vi "Create Command String.vi"(8 "error in (no error)":errorcluster, 11 "Channel Params":T1={"channel"=enum."2", "gain"=enum."10x", "input"=enum."DIFF", "shunt"=enum."Open", "couple"=enum."DC", "filter"=enum."ON"}) -> (0 "error out":errorcluster, 3 "Command string":string)   [LabVIEW 2019, in "KH7008.lvlib"]
uses:
  KH7008.lvlib
  typedefs/channelProperties--Cluster.ctl
  typedefs/channel--enum.ctl
  typedefs/gain--enum.ctl
  typedefs/input--enum.ctl
  typedefs/shunt--enum.ctl
  typedefs/couple--enum.ctl
  typedefs/filter--enum.ctl
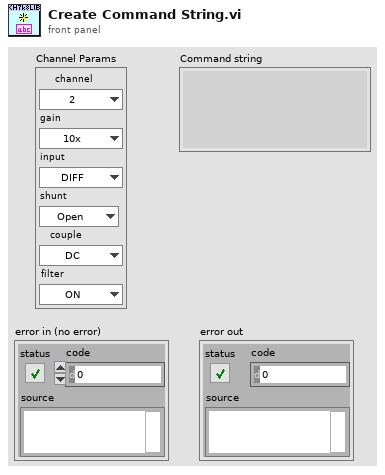
[diagram p1: front panel]
types:
  T1 = typedef "KH7008.lvlib/channelProperties--Cluster.ctl" = cluster{"channel":T2, "gain":T3, "input":T4, "shunt":T5, "couple":T6, "filter":T7}
  T2 = typedef "KH7008.lvlib/channel--enum.ctl" = enum16{"1", "2", "3", "4", "5", "6", "7", "8"}
  T3 = typedef "KH7008.lvlib/gain--enum.ctl" = enum16{"1x", "10x", "100x", "1000x"}
  T4 = typedef "KH7008.lvlib/input--enum.ctl" = enum16{"OFF", "SE+", "SE-", "DIFF"}
  T5 = typedef "KH7008.lvlib/shunt--enum.ctl" = enum16{"Open", "50", "500", "5k", "50k", "10M"}
  T6 = typedef "KH7008.lvlib/couple--enum.ctl" = enum16{"AC", "DC"}
  T7 = typedef "KH7008.lvlib/filter--enum.ctl" = enum16{"OFF", "ON"}
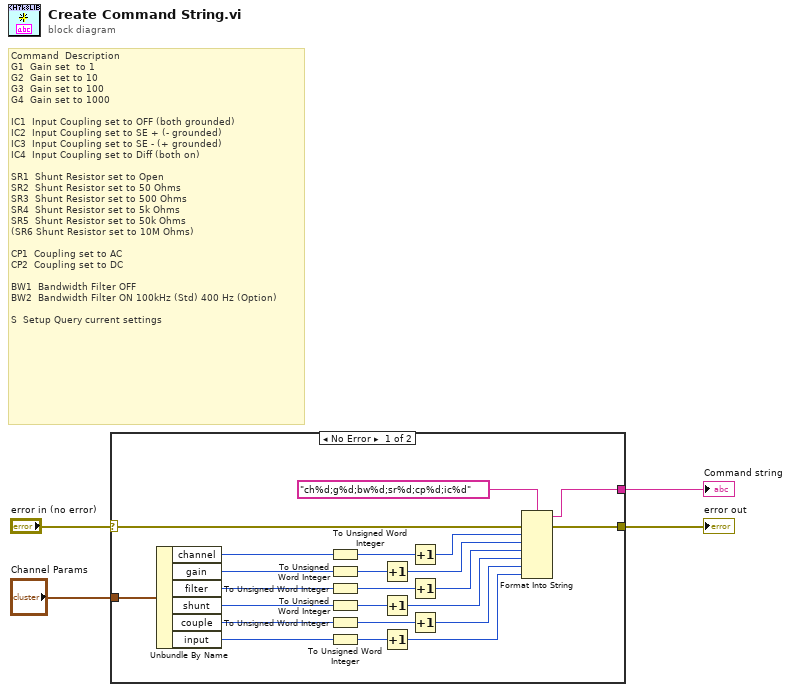
[diagram p0: block diagram]
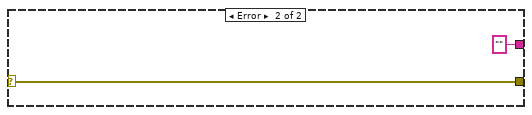
[diagram p2: hidden frame]
diagram:
  # "Command  Description \nG1  Gain set  to 1 \nG2  Gain set to 10 \nG3  Gain set to 100 \nG4  Gain set to 1000 \n   \nIC1  Input Coupling set to OFF (both grounded) \nIC2  Input Coupling set to SE + (- grounded) \nIC3  Input Coupling set to SE - (+ grounded) \nIC4  Input Coupling set to Diff (both on) \n   \nSR1  Shunt Resistor set to Open \nSR2  Shunt Resistor set to 50 Ohms \nSR3  Shunt Resistor set to 500 Ohms \nSR4  Shunt Resistor set to 5k Ohms \nSR5  Shunt Resistor set to 50k Ohms \n(SR6 Shunt Resistor set to 10M Ohms)\n   \nCP1  Coupling set to AC \nCP2  Coupling set to DC \n   \nBW1  Bandwidth Filter OFF \nBW2  Bandwidth Filter ON 100kHz (Std) 400 Hz (Option)\n   \nS  Setup Query current settings"
  n1 = case shown="No Error" "error in (no error)" {
    selector: "error in (no error)" -> [w25 w29]
    tunnel: [w27 ""] -> w4
    tunnel: [w26 w29] -> w3
    tunnel: "Channel Params" -> [w11 _]
    frame No Error {
      n2 = Unbundle By Name(w11) -> ("channel"=w10:T2, "gain"=w9:T3, "filter"=w8:T7, "shunt"=w7:T5, "couple"=w6:T6, "input"=w5:T4)
      n3 = To Unsigned Word Integer(number=w10) -> (unsigned 16bit integer=w19:u16)
      n4 = To Unsigned Word Integer(number=w9) -> (unsigned 16bit integer=w20:u16)
      n5 = To Unsigned Word Integer(number=w8) -> (unsigned 16bit integer=w21:u16)
      n6 = To Unsigned Word Integer(number=w7) -> (unsigned 16bit integer=w22:u16)
      n7 = To Unsigned Word Integer(number=w6) -> (unsigned 16bit integer=w23:u16)
      n8 = To Unsigned Word Integer(number=w5) -> (unsigned 16bit integer=w24:u16)
      n9 = Increment(x=w20) -> (x+1=w14:u16)
      n10 = Increment(x=w22) -> (x+1=w15:u16)
      n11 = Increment(x=w24) -> (x+1=w18:u16)
      n12 = Increment(x=w19) -> (x+1=w13:u16)
      n13 = Increment(x=w21) -> (x+1=w16:u16)
      n14 = Increment(x=w23) -> (x+1=w17:u16)
      n15 = Format Into String(format string="ch%d;g%d;bw%d;sr%d;cp%d;ic%d", error in=w25, w13, w14, w16, w15, w17, w18) -> (resulting string=w27:string, error out=w26:errorcluster)  [unwired: 1 in]
    }
    frame Error {
    }
  }
  "Command string" <- w4
  "error out" <- w3
